vi "CRYChannel separate buffer array.vi"(10 "N channels":i32, 11 "Buffer array in":i32[](array[numeric])) -> (1 "First right channel":i32[](array[numeric]), 2 "First left channel":i32[](array[numeric]), 3 "Channel-separated arrays":i32[][](array[numeric]))   [LabVIEW 2013]
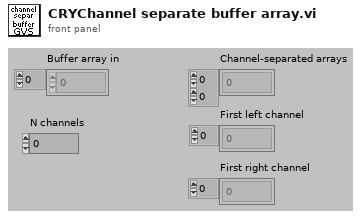
[diagram p1: front panel]
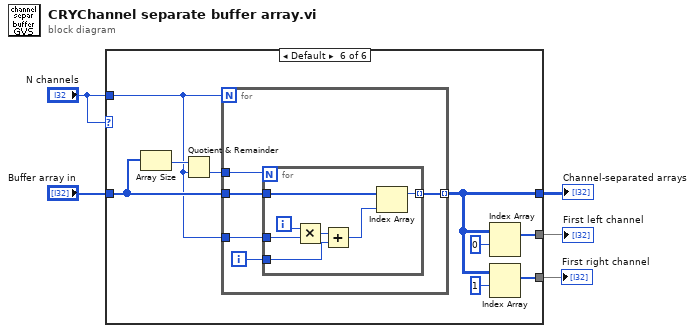
[diagram p0: block diagram]
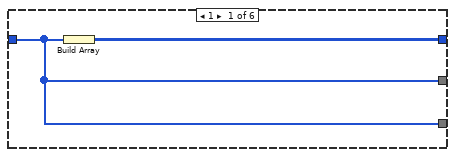
[diagram p2: hidden frame]
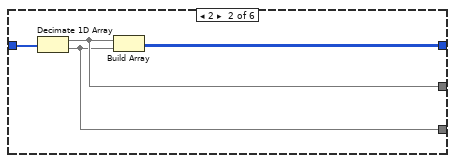
[diagram p3: hidden frame]
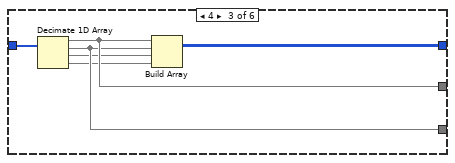
[diagram p4: hidden frame]
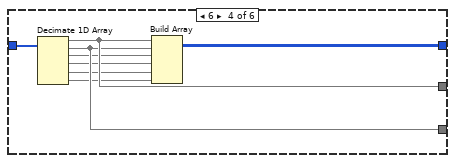
[diagram p5: hidden frame]
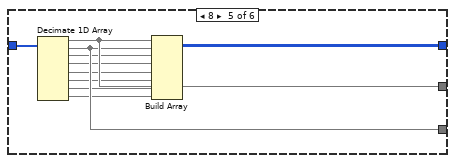
[diagram p6: hidden frame]
diagram:
  n1 = case shown="Default" "N channels" {
    tunnel: "Buffer array in" -> [w6 w11 w17 w25 w35 w42]
    tunnel: [w7 w10 w16 w24 w34 w36] -> w4
    tunnel: [w6 w9 w15 w23 w33 w38] -> w3
    tunnel: [w6 w8 w14 w22 w32 w37] -> w2
    tunnel: "N channels" -> [_ _ _ _ _ w41]
    frame 1 {
      n2 = Build Array(w6) -> (w7:i32[][])
    }
    frame 2 {
      n3 = Decimate 1D Array(w11) -> (w9:i32[], w8:i32[])
      n4 = Build Array(w9, w8) -> (w10:i32[][])
    }
    frame 4 {
      n5 = Decimate 1D Array(w17) -> (w15:i32[], w14:i32[], w13:i32[], w12:i32[])
      n6 = Build Array(w15, w14, w13, w12) -> (w16:i32[][])
    }
    frame 6 {
      n7 = Decimate 1D Array(w25) -> (w23:i32[], w22:i32[], w21:i32[], w20:i32[], w19:i32[], w18:i32[])
      n8 = Build Array(w23, w22, w21, w20, w19, w18) -> (w24:i32[][])
    }
    frame 8 {
      n9 = Decimate 1D Array(w35) -> (w33:i32[], w32:i32[], w31:i32[], w30:i32[], w29:i32[], w28:i32[], w27:i32[], w26:i32[])
      n10 = Build Array(w33, w32, w31, w30, w29, w28, w27, w26) -> (w34:i32[][])
    }
    frame Default {
      n11 = Array Size(array=w42) -> (size(s)=w44:i32)
      n12 = Quotient & Remainder(x=w44, y=w41) -> (floor(x/y)=w43:i32)  [unwired: 1 out]
      n13 = for {
        N: w41 -> [_]
        tunnel: w43 -> [w49]
        tunnel: w42 -> [w48]
        tunnel: w41 -> [w47]
        tunnel: [w45] -> w36 mode=indexing
        i -> [w46]
        n14 = for {
          N: w49 -> [_]
          tunnel: w48 -> [w56]
          tunnel: w47 -> [w55]
          tunnel: w46 -> [w53]
          tunnel: [w50] -> w45 mode=indexing
          i -> [w54]
          n15 = Multiply(x=w54, y=w55) -> (x*y=w52:i32)
          n16 = Add(x=w52, y=w53) -> (x+y=w51:i32)
          n17 = Index Array(array=w56, index=w51) -> (element=w50:i32)
        }
      }
      n18 = Index Array(array=w36, index (row)=0 ("Index")) -> (element=w38:i32[])  [unwired: 1 in]
      n19 = Index Array(array=w36, index (row)=1 ("Index")) -> (element=w37:i32[])  [unwired: 1 in]
    }
  }
  "Channel-separated arrays" <- w4
  "First left channel" <- w3
  "First right channel" <- w2
